vi "configuration_write.vi"(8 "error in (no error)":errorcluster, 10 "configuration":variant, 11 "lv-builder-l3 in":refnum<class "lv-builder-l3.lvclass">) -> (0 "error out":errorcluster, 3 "lv-builder-l3 out":refnum<class "lv-builder-l3.lvclass">)   [LabVIEW 2015, in "lv-builder-l3.lvlib" / "lv-builder-l3.lvclass"]
uses:
  lv-builder-l3.lvclass
  lv-builder-l3.lvclass/lv-builder-l3.ctl
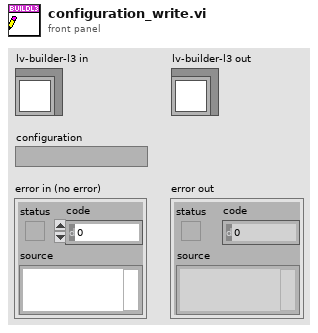
[diagram p1: front panel]
types:
  T1 = typedef "lv-builder-l3.lvlib/configuration.ctl" = cluster{"l3_archive_file_path":string}
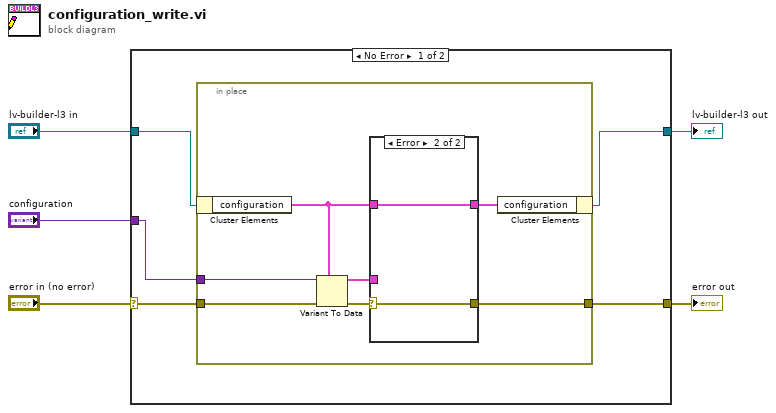
[diagram p0: block diagram]
diagram:
  n1 = case shown="No Error" "error in (no error)" {
    selector: "error in (no error)" -> [w8 w22]
    tunnel: [w6 w22] -> w4
    tunnel: [w9 w23] -> w2
    tunnel: "lv-builder-l3 in" -> [w10 w23]
    tunnel: "configuration" -> [w7 _]
    frame No Error {
      n2 = in-place {
        in-place-border: w8 -> [w17]
        in-place-border: w7 -> [w16]
        in-place-border: [w13] -> w6
        n3 = in-place-cluster #1(w10) -> ("configuration"=w12:T1)
        n4 = Variant To Data(error in=w17, type=w12, Variant=w16) -> (data=w15:T1, error out=w14:errorcluster)
        n5 = case shown="Error" w14 {
          selector: w14 -> [w19 w20]
          tunnel: w15 -> [w18 _]
          tunnel: [w19 w20] -> w13
          tunnel: w12 -> [_ w21]
          tunnel: [w18 w21] -> w11
          frame No Error {
          }
          frame Error {
          }
        }
        n6 = in-place-cluster #1("configuration"=w11) -> (w9:refnum<class "lv-builder-l3.lvclass">)
      }
    }
    frame Error {
    }
  }
  "error out" <- w4
  "lv-builder-l3 out" <- w2
